vi "MAP_FGV_IN.vi"(8 "error in (no error)":errorcluster, 9 "DOs":bool[](array[boolean]), 11 "Relay_ENUM_IN":T1[](array[typedef])) -> (0 "error out":errorcluster, 2 "DOs_out":bool[](array[boolean]), 3 "Relay_ENUM_IN 2":T1[](array[typedef]))   [LabVIEW 2024, in "ADAM_DI.lvlib"]
uses:
  ADAM_DI.lvlib
  Relay_enum_IN.ctl
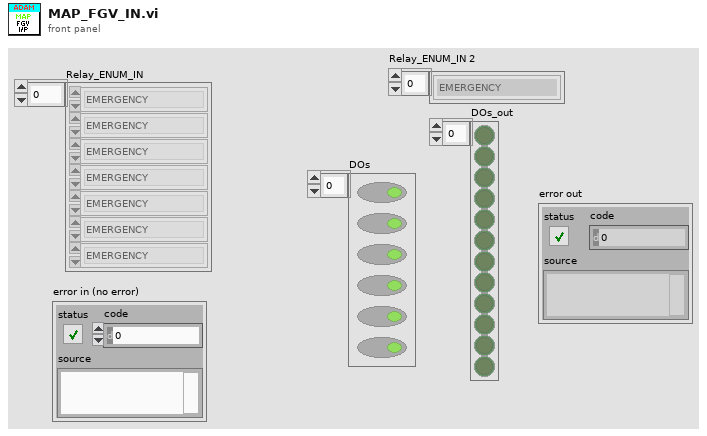
[diagram p1: front panel]
types:
  T1 = typedef "ADAM_DI.lvlib/Relay_enum_IN.ctl" = enum16{"EMERGENCY", "CONTROL ON", "START DUT 1", "START DUT 2", "STOP DUT 1", "STOP DUT 2", "PPS DUT 1", "PPS DUT 2", "REED CYL UP DUT 1", "REED CYL DOWN DUT 1", "REED CYL UP DUT 2", "REED CYL DOWN DUT 2", "LIGHT CURTAIN"}
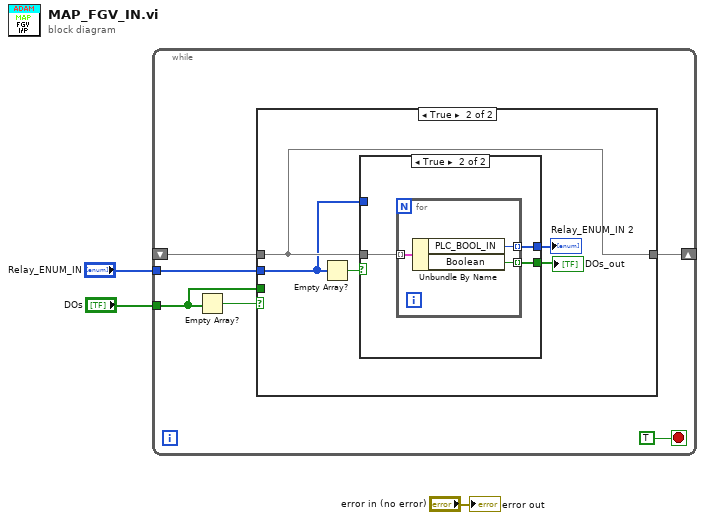
[diagram p0: block diagram]
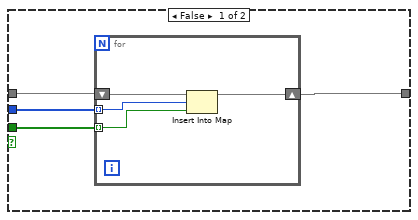
[diagram p2: hidden frame]
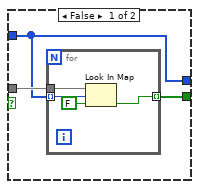
[diagram p3: hidden frame]
diagram:
  n1 = while {
    tunnel: "DOs" -> [w6]
    tunnel: "Relay_ENUM_IN" -> [w7]
    shift-right: [w5] -> _
    shift-left: _ -> [w4]
    stop <- TRUE stop-if-true
    n2 = Empty Array?(array=w6) -> (empty?=w8:bool)
    n3 = case shown="True" w8 {
      tunnel: w7 -> [w13 w20]
      tunnel: w6 -> [w12 _]
      tunnel: [w11 w21] -> w5
      tunnel: w4 -> [w10 w21]
      frame False {
        n4 = for {
          tunnel: w13 -> [w17] mode=indexing
          tunnel: w12 -> [w16] mode=indexing
          shift-right: [w15] -> w11
          shift-left: w10 -> [w14]
          n5 = Insert Into Map(map in=w14, key=w17, value=w16) -> (map out=w15:map{T1, bool})  [unwired: 2 out]
        }
      }
      frame True {
        n6 = Empty Array?(array=w20) -> (empty?=w22:bool)
        n7 = case shown="True" w22 {
          tunnel: w21 -> [w25 w32]
          tunnel: [w23 w31] -> w19
          tunnel: [w24 w30] -> w18
          tunnel: w20 -> [w23 _]
          frame False {
            n8 = for {
              tunnel: w25 -> [w29]
              tunnel: [w28] -> w24 mode=indexing
              tunnel: w23 -> [w27] mode=indexing
              n9 = Look In Map(map=w29, key=w27, default value=FALSE) -> (value=w28:bool)  [unwired: 1 out]
            }
          }
          frame True {
            n10 = for {
              tunnel: w32 -> [w35] mode=indexing
              tunnel: [w34] -> w31 mode=indexing
              tunnel: [w33] -> w30 mode=indexing
              n11 = Unbundle By Name(w35) -> ("PLC_BOOL_IN"=w34:T1, "Boolean"=w33:bool)
            }
          }
        }
        "Relay_ENUM_IN 2" <- w19
        "DOs_out" <- w18
      }
    }
  }
  "error out" <- "error in (no error)"
